vi "stop_usb6343.vi"(8 "错误输入（无错误）":errorcluster, 11 "msg interface":T1) -> (0 "错误输出":errorcluster)   [LabVIEW 2013]
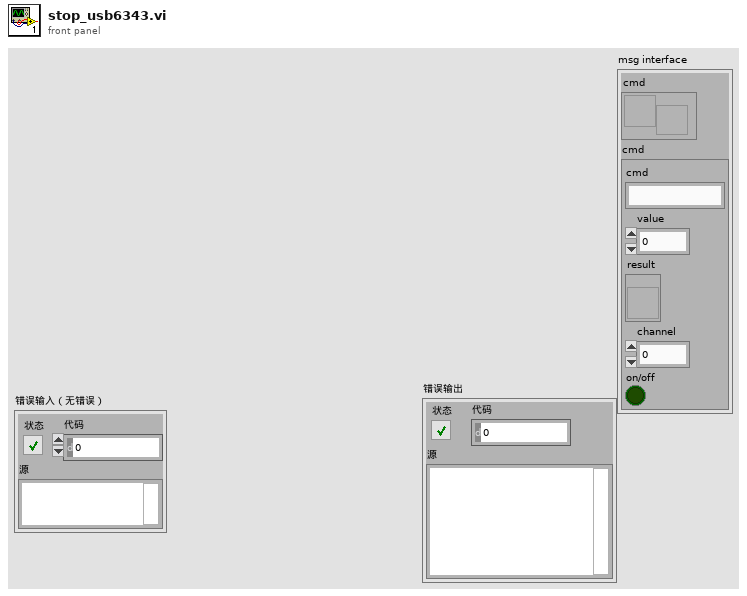
[diagram p1: front panel]
types:
  T1 = cluster{"cmd":refnum<user-event>, "cmd":cluster{"cmd":string, "value":dbl, "result ":refnum<vi>, "channel":i32, "on/off":bool}}
  T2 = cluster{"cmd":string, "value":dbl, "result ":refnum<vi>, "channel":i32, "on/off":bool}
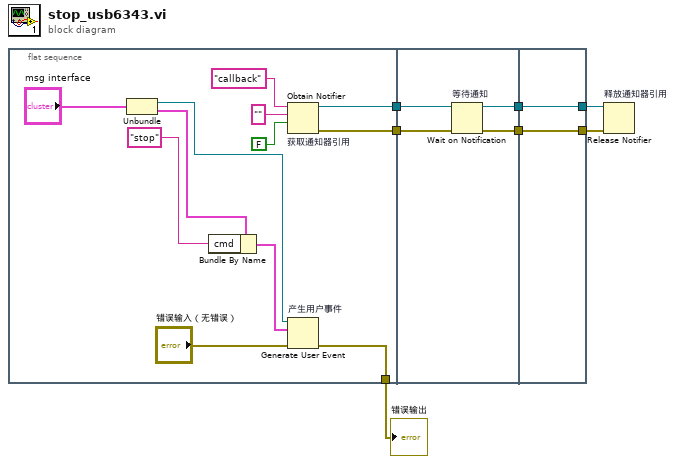
[diagram p0: block diagram]
diagram:
  n1 = flat-sequence {
    tunnel: [w11] -> w7
    tunnel: [w9] -> w6
    tunnel: [w8] -> w5
    tunnel: w7 -> [w23]
    tunnel: w6 -> [w22]
    tunnel: [w21] -> w4
    tunnel: [w20] -> w2
    tunnel: w4 -> [w25]
    tunnel: [w25] -> w3
    tunnel: w2 -> [w24]
    tunnel: [w24] -> w1
    frame #0 {
      n2 = Unbundle("msg interface") -> ("cmd"=w16:refnum<user-event>, "cmd"=w15:T2)
      n3 = Bundle By Name(cluster=w15, "cmd"="stop") -> (w19:T2)
      n4 = Obtain Notifier "获取通知器引用"(name (unnamed)="callback" ("名称（未命名）"), notification data type="", create if not found? (T)=FALSE ("如未找到是否创建？(T)")) -> (notifier out=w11:refnum<notifier>, error out=w9:errorcluster)  [unwired: 1 in, 1 out]
      n5 = Generate User Event "产生用户事件"(user event=w16, event data cluster=w19, error in="错误输入（无错误）") -> (error out=w8:errorcluster)  [unwired: 1 in, 1 out]
    }
    frame #1 {
      n6 = Wait on Notification "等待通知"(notifier=w23, error in (no error)=w22) -> (notifier out=w21:refnum<notifier>, error out=w20:errorcluster)  [unwired: 2 in, 2 out]
    }
    frame #2 {
    }
  }
  n7 = Release Notifier "释放通知器引用"(notifier=w3, error in (no error)=w1) -> ()  [unwired: 1 in, 3 out]
  "错误输出" <- w5
